vi "Get DIO Lines.vi"(8 "error in (no error)":errorcluster, 11 "RIO Target in":refnum<class "RIO Target.lvclass">) -> (0 "error out":errorcluster, 2 "DIO Lines":string[](array[string]), 3 "RIO Target out":refnum<class "RIO Target.lvclass">)   [LabVIEW 2014, in "RIO Target.lvclass"]
uses:
  RIO Target.lvclass
  RIO Target.lvclass/RIO Target.ctl
  <vilib>/NI/Configuration Framework/serializable configuration/read metadata property.vi
  <vilib>/xml/Load XML File.vi
  <vilib>/xml/Close Reference(Node).vi
  <vilib>/xml/Close Reference(NNMap).vi
  <vilib>/xml/Close Reference(NdList).vi
  <vilib>/xml/NI_XML.lvlib
  <resource>/objmgr/DOMUserDefRef.rc
  RIO Target Configuration/RIO Target Configuration.lvclass
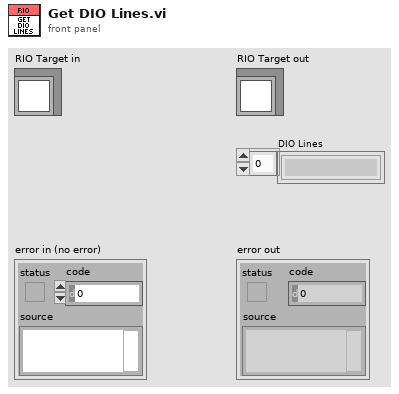
[diagram p1: front panel]
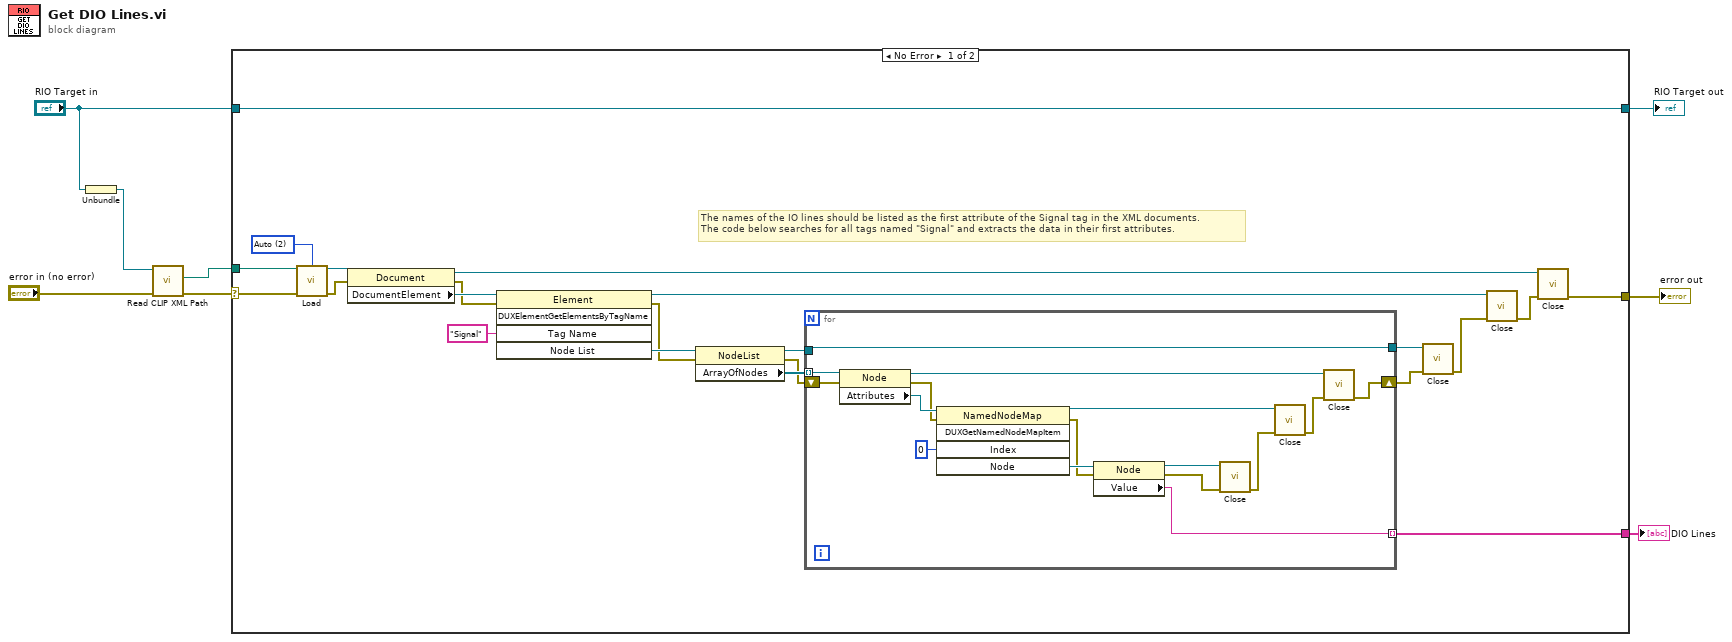
[diagram p0: block diagram]
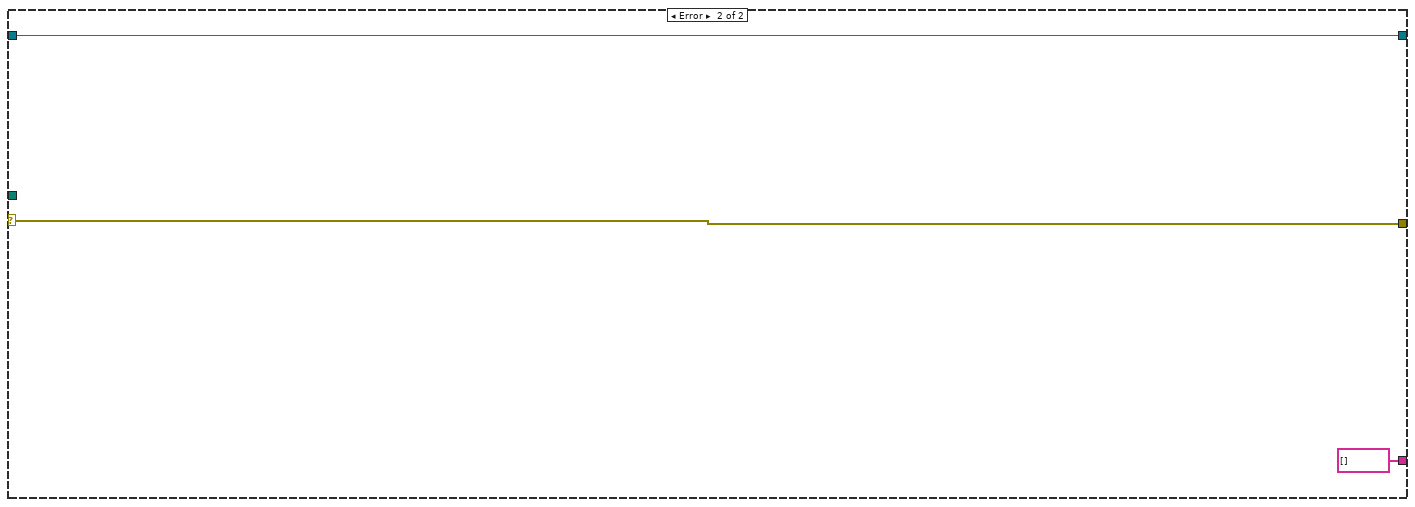
[diagram p2: hidden frame]
diagram:
  n1 = Unbundle("RIO Target in") -> (w1:refnum<class "RIO Target Configuration.lvclass">)
  n2 = call "Read CLIP XML Path.vi"("error in (no error)"="error in (no error)", "RIO Target Configuration in"=w1) -> ("error out"=w4:errorcluster, "CLIP XML Path"=w3:path)  [unwired: 7 in, 1 out]
  n3 = case shown="No Error" w4 {
    selector: w4 -> [w12 w49]
    tunnel: [w11 w49] -> w7
    tunnel: [w30 w48] -> w8
    tunnel: "RIO Target in" -> [w30 w48]
    tunnel: w3 -> [w9 _]
    tunnel: [w10 string[] []] -> w6
    frame No Error {
      w29 = 2 items=["Never", "Always", "Auto"] ("validate on load (Auto)")
      # "The names of the IO lines should be listed as the first attribute of the Signal tag in the XML documents. \nThe code below searches for all tags named \"Signal\" and extracts the data in their first attributes."
      n4 = call-poly <vilib>:"Load.vi"("path to XML document"=w9, "validate on load (Auto)"=w29, "error in (no error)"=w12) -> ("DOM document out"=w28:refnum<k20>, "error out"=w25:errorcluster)  [unwired: 10 in, 1 out]
      n5 = property class="Document"(reference=w28, error in=w25) -> (reference out=w19:refnum<k20>, error out=w24:errorcluster, "DocumentElement"=w27:refnum<k20>)
      n6 = invoke class="Element" method="DUXElementGetElementsByTagName"(reference=w27, error in=w24, "Tag Name"="Signal") -> (reference out=w20:refnum<k20>, error out=w18:errorcluster, "Node List"=w23:refnum<k20>)  [unwired: 2 in, 2 out]
      n7 = property class="NodeList"(reference=w23, error in=w18) -> (reference out=w17:refnum<k20>, error out=w16:errorcluster, "ArrayOfNodes"=w22:refnum<k20>[])
      n8 = for {
        tunnel: w22 -> [w33] mode=indexing
        tunnel: w17 -> [w34]
        shift-right: [w31] -> w15
        shift-left: w16 -> [w32]
        tunnel: [w43] -> w10 mode=indexing
        tunnel: [w34] -> w13
        n9 = property class="Node"(reference=w33, error in=w32) -> (reference out=w39:refnum<k20>, error out=w45:errorcluster, "Attributes"=w46:refnum<k20>)
        n10 = invoke class="NamedNodeMap" method="DUXGetNamedNodeMapItem"(reference=w46, error in=w45, "Index"=0) -> (reference out=w38:refnum<k20>, error out=w37:errorcluster, "Node"=w44:refnum<k20>)  [unwired: 2 in, 2 out]
        n11 = property class="Node"(reference=w44, error in=w37) -> (reference out=w36:refnum<k20>, error out=w42:errorcluster, "Value"=w43:string)
        n12 = call-poly <vilib>:"Close.vi"("error in (no error)"=w42, "node"=w36) -> ("error out"=w41:errorcluster)  [unwired: 7 out]
        n13 = call-poly <vilib>:"Close.vi"("error in (no error)"=w41, "named node map"=w38) -> ("error out"=w40:errorcluster)  [unwired: 7 out]
        n14 = call-poly <vilib>:"Close.vi"("error in (no error)"=w40, "node"=w39) -> ("error out"=w31:errorcluster)  [unwired: 7 out]
      }
      n15 = call-poly <vilib>:"Close.vi"("error in (no error)"=w15, "node list"=w13) -> ("error out"=w14:errorcluster)  [unwired: 7 out]
      n16 = call-poly <vilib>:"Close.vi"("error in (no error)"=w14, "node"=w20) -> ("error out"=w21:errorcluster)  [unwired: 7 out]
      n17 = call-poly <vilib>:"Close.vi"("error in (no error)"=w21, "node"=w19) -> ("error out"=w11:errorcluster)  [unwired: 7 out]
    }
    frame Error {
    }
  }
  "error out" <- w7
  "RIO Target out" <- w8
  "DIO Lines" <- w6
